vi "Read Processes.vi"(4 "Error In":errorcluster, 6 "Launch Condition":T1, 7 "DB_ADO in":refnum<class "Config Data_DB_ADO.lvclass">) -> (0 "Error Out":errorcluster, 2 "Processes to Launch":T2[](array[typedef]), 3 "DB_ADO out":refnum<class "Config Data_DB_ADO.lvclass">)   [LabVIEW 2020, in "Config Data.lvlib" / "Config Data_DB_ADO.lvclass"]
uses:
  Config Data_DB_ADO.lvclass
  C:/Users/Fred Guo/Desktop/Release 19/_libraries/Config Data/DB/Config Data_DB.lvclass
  typedefs/Process Launch Data.ctl
  typedefs/Process Type.ctl
  typedefs/Launch Location.ctl
  toolbox/ADO Database Drivers/ADO Database Drivers.lvlib
  Config Data_DB.lvclass
  Config Data.lvclass
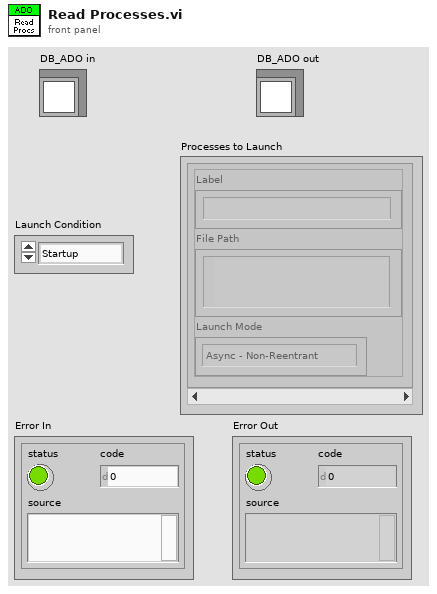
[diagram p1: front panel]
types:
  T1 = typedef "Config Data.lvlib/Config Data.lvclass/Launch Location.ctl" = enum16{"Startup", "Subpanels"}
  T2 = typedef "Config Data.lvlib/Config Data.lvclass/Process Launch Data.ctl" = cluster{"Label":string, "File Path":path, "Launch Mode":T3}
  T3 = typedef "Config Data.lvlib/Config Data.lvclass/Process Type.ctl" = enum16{"Async - Non-Reentrant", "Async - Reentrant", "Run Method - Non-Reentrant", "Run Method - Reentrant"}
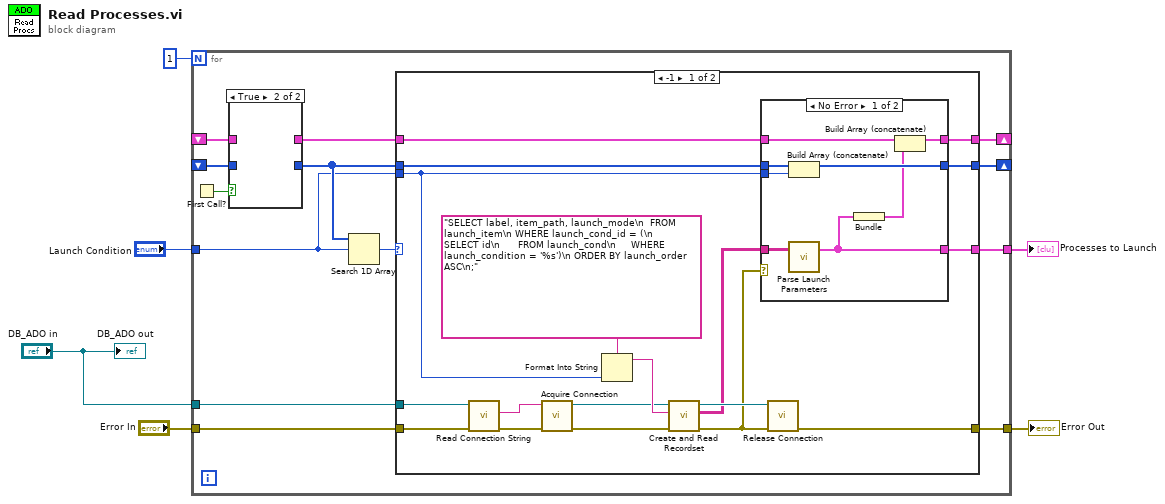
[diagram p0: block diagram]
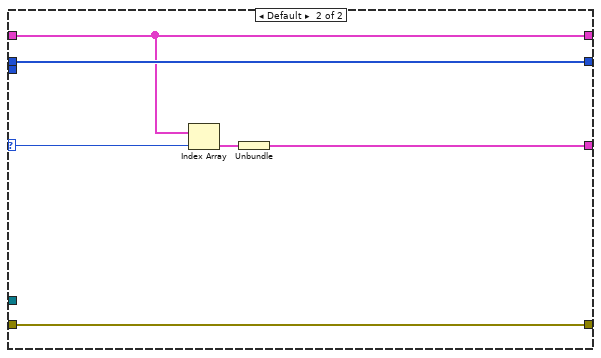
[diagram p3: hidden frame]
diagram:
  n1 = for {
    N: 1 -> [_]
    tunnel: [w19] -> w4
    tunnel: "Error In" -> [w14]
    shift-right: [w16] -> _
    shift-left: _ -> [w10]
    shift-right: [w18] -> _
    shift-left: _ -> [w12]
    tunnel: [w15] -> w2
    tunnel: "Launch Condition" -> [w7]
    tunnel: "DB_ADO in" -> [w8]
    n2 = First Call?() -> (First Call?: T/F=w9:bool)
    n3 = case shown="True" w9 {
      tunnel: [w55 _] -> w13
      tunnel: w12 -> [w55 _]
      tunnel: [w54 _] -> w11
      tunnel: w10 -> [w54 _]
      frame False {
      }
      frame True {
      }
    }
    n4 = Search 1D Array(1D array=w11, element=w7) -> (index of element=w17:i32)  [unwired: 1 in]
    n5 = case shown="-1" w17 {
      selector: w17 -> [_ w51]
      tunnel: w14 -> [w25 w53]
      tunnel: [w36 w53] -> w19
      tunnel: [w32 w50] -> w18
      tunnel: w13 -> [w33 w50]
      tunnel: [w30 w52] -> w16
      tunnel: w11 -> [w31 w52]
      tunnel: w7 -> [w20 _]
      tunnel: [w28 w48] -> w15
      tunnel: w8 -> [w23 _]
      frame -1 {
        n6 = call "Read Connection String.vi"("Error In"=w25, "DB In"=w23) -> ("Error Out"=w24:errorcluster, "Connection String"=w26:string)  [unwired: 3 in, 1 out]
        n7 = call "Acquire Connection.vi"("error in (no error)"=w24, "Connection String"=w26) -> ("error out"=w21:errorcluster, "Connection"=w22:refnum<k7>)  [unwired: 3 in, 1 out]
        n8 = Format Into String(format string="SELECT label, item_path, launch_mode\n  FROM launch_item\n WHERE launch_cond_id = (\n    SELECT id\n      FROM launch_cond\n     WHERE launch_condition = '%s')\n ORDER BY launch_order ASC\n;", w20) -> (resulting string=w35:string)  [unwired: 2 in, 1 out]
        n9 = call "Create and Read Recordset.vi"("error in (no error)"=w21, "Source"=w35, "Connection In"=w22) -> ("error out"=w34:errorcluster, "DB Data"=w29:string[][], "Connection Out"=w37:refnum<k7>)  [unwired: 2 in, 2 out]
        n10 = case shown="No Error" w34 {
          tunnel: w33 -> [w42 w47]
          tunnel: [w41 w47] -> w32
          tunnel: w31 -> [w45 w46]
          tunnel: [w44 w46] -> w30
          tunnel: w20 -> [w43 _]
          tunnel: w29 -> [w38 _]
          tunnel: [w39 _] -> w28
          frame No Error {
            n11 = Build Array (concatenate)(w45, w43) -> (w44:T1[])
            n12 = call "Parse Launch Parameters.vi"("DB Data"=w38) -> ("Processes to Launch"=w39:T2[])  [unwired: 2 in]
            n13 = Bundle("Processes to Launch"=w39) -> (w40:cluster{"Processes to Launch":T2[]})  [unwired: 1 in]
            n14 = Build Array (concatenate)(w42, w40) -> (w41:cluster{"Processes to Launch":T2[]}[])
          }
          frame Error {
          }
        }
        n15 = call "Release Connection.vi"("error in"=w34, "Connection"=w37) -> ("error out"=w36:errorcluster)  [unwired: 5 in]
      }
      frame Default {
        n16 = Index Array(array=w50, index=w51) -> (element=w49:cluster{"Processes to Launch":T2[]})
        n17 = Unbundle(w49) -> ("Processes to Launch"=w48:T2[])
      }
    }
  }
  "Error Out" <- w4
  "Processes to Launch" <- w2
  "DB_ADO out" <- "DB_ADO in"
